vi "ReadEditToleranceOverrideJSON.vi"(8 "error in":errorcluster, 9 "Algo Override\nJSON Variant in":variant, 10 "Read Edit Tolerance \nOverride JSON":path=path "C:/Users/raakeshs/Desktop/GTRON/JSONs/DeafultJSON_Final.json", 11 "Part Name":string) -> (0 "error out":errorcluster, 3 "Cluster":T1)   [LabVIEW 2019, in "ZenGage v3.0 UI.lvclass"]
uses:
  ZenGage v3.0 UI.lvclass
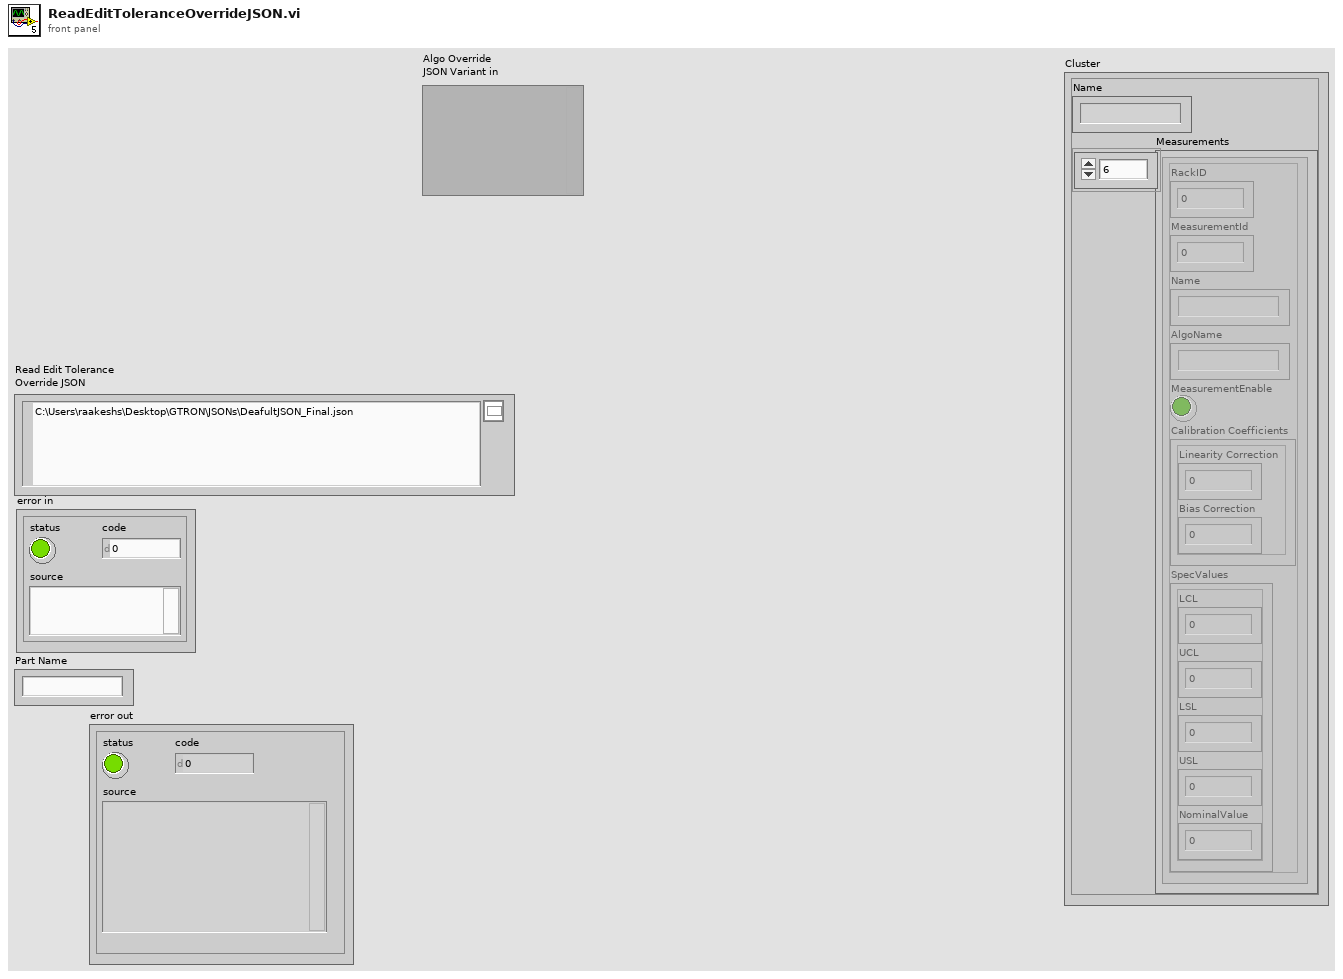
[diagram p1: front panel]
types:
  T1 = cluster{"Name":string, "Measurements":cluster{"RackID":i32, "MeasurementId":i32, "Name":string, "AlgoName":string, "MeasurementEnable":bool, "Calibration Coefficients":cluster{"Linearity Correction":dbl, "Bias Correction":dbl}, "SpecValues":cluster{"LCL":dbl, "UCL":dbl, "LSL":dbl, "USL":dbl, "NominalValue":dbl}}[]}
  T2 = typedef "ZenGage v3.0 UI.lvclass/Algo(Override)_CoeffficientsIncluded.ctl" = cluster{"AlgoParameters":cluster{"PartsList":cluster{"Name":string, "Measurements":cluster{"RackID":dbl, "MeasurementId":dbl, "Name":string, "AlgoName":string, "MeasurementEnable":bool, "UserCalibCoefficients":cluster{"UserCorrectionLinearityCoeff":dbl, "UserCorrectionBiasCoeff":dbl}, "SpecValues":cluster{"LCL":dbl, "UCL":dbl, "LSL":dbl, "USL":dbl, "NominalValue":dbl}}[]}[]}}
  T3 = cluster{"Name":string, "Measurements":cluster{"RackID":dbl, "MeasurementId":dbl, "Name":string, "AlgoName":string, "MeasurementEnable":bool, "UserCalibCoefficients":cluster{"UserCorrectionLinearityCoeff":dbl, "UserCorrectionBiasCoeff":dbl}, "SpecValues":cluster{"LCL":dbl, "UCL":dbl, "LSL":dbl, "USL":dbl, "NominalValue":dbl}}[]}[]
  T4 = cluster{"Name":string, "Measurements":cluster{"RackID":dbl, "MeasurementId":dbl, "Name":string, "AlgoName":string, "MeasurementEnable":bool, "UserCalibCoefficients":cluster{"UserCorrectionLinearityCoeff":dbl, "UserCorrectionBiasCoeff":dbl}, "SpecValues":cluster{"LCL":dbl, "UCL":dbl, "LSL":dbl, "USL":dbl, "NominalValue":dbl}}[]}
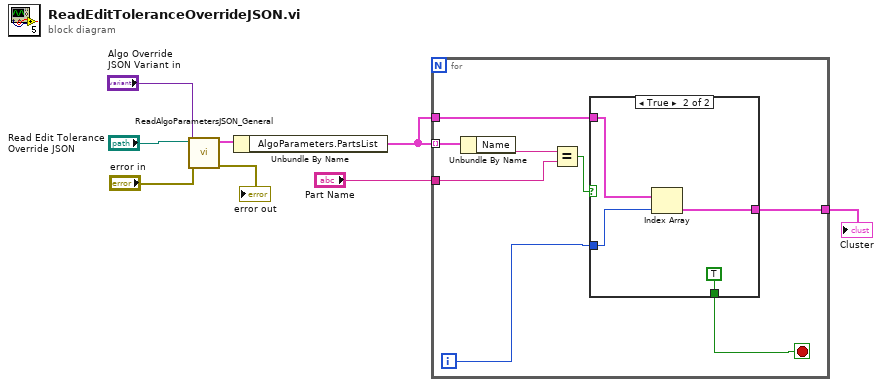
[diagram p0: block diagram]
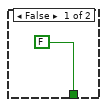
[diagram p2: hidden frame]
diagram:
  n1 = call "ReadAlgoParametersJSON_General.vi"("error in"="error in", "Algo Override\nJSON Variant in"="Algo Override\nJSON Variant in", "Read Edit Tolerance \nOverride JSON"="Read Edit Tolerance \nOverride JSON") -> ("error out"=→"error out":errorcluster, "ZenGage v3.0 UI.lvclass:Algo(Override)_CoeffficientsIncluded"=w6:T2)  [unwired: 6 in, 1 out]
  n2 = Unbundle By Name(w6) -> ("AlgoParameters.PartsList"=w4:T3)
  n3 = for {
    tunnel: w4 -> [w16] mode=indexing
    tunnel: "Part Name" -> [w14]
    tunnel: w4 -> [w11]
    tunnel: [w10] -> w1
    i -> [w12]
    stop <- w9 stop-if-true
    n4 = Unbundle By Name(w16) -> ("Name"=w15:string)
    n5 = Equal?(x=w15, y=w14) -> (x = y?=w13:bool)
    n6 = case shown="True" w13 {
      tunnel: w12 -> [_ w20]
      tunnel: w11 -> [_ w21]
      tunnel: [_ w19] -> w10
      tunnel: [FALSE TRUE] -> w9
      frame False {
      }
      frame True {
        n7 = Index Array(array=w21, index=w20) -> (element=w19:T4)
      }
    }
  }
  "Cluster" <- w1
